vi "Read PDP Values.vi"() -> (3 "all currents (A)":dbl[](array[numeric]))   [LabVIEW 2018]
panel:
  out "current (A)":dbl
  in  "Tare Currents?":bool
  in  "PDP Channel":i32
  in  "Power Distribution Panel (0)":u8
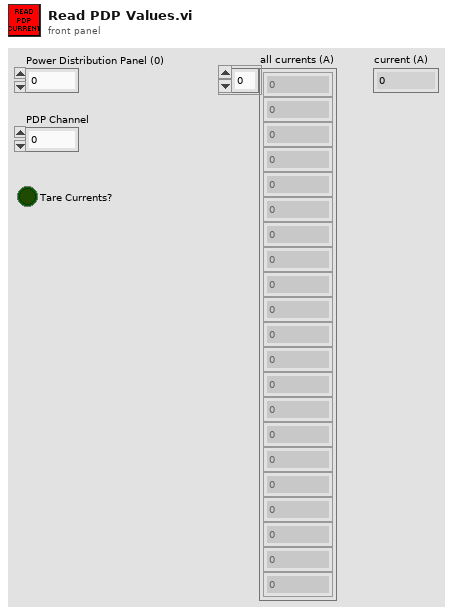
[diagram p1: front panel]
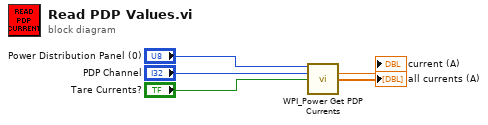
[diagram p0: block diagram]
diagram:
  n1 = call <vilib>:"WPI_Power Get PDP Currents.vi"("Power Distribution Panel (0)"="Power Distribution Panel (0)", "PDP Channel"="PDP Channel", "Tare Currents?"="Tare Currents?") -> ("current (A)"=→"current (A)":dbl, "all currents (A)"=→"all currents (A)":dbl[])  [unwired: 10 in, 1 out]
